vi "_TEST Templates.vi"(4 "error in (no error)":errorcluster) -> (0 "error out":errorcluster)   [LabVIEW 2011]
uses:
  Template Record.ctl
  <vilib>/addons/internet/utils/keyedarr.llb/Keyed Array.ctl
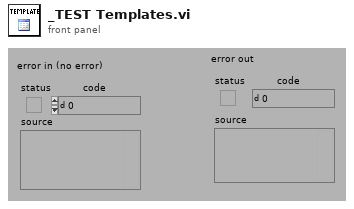
[diagram p1: front panel]
types:
  T1 = typedef "Keyed Array.ctl" = cluster{"keys":string[], "values":string[]}
  T2 = typedef "Template Record.ctl" = cluster{"ixTemplate":i32, "sxTemplateId":string, "sDescription":string, "sCreator":string, "tCreationDate":timestamp, "sModifier":string, "tModifiedDate":timestamp, "sType":string, "sStyle":string, "sFormat":string, "dWidth":dbl, "dHeight":dbl, "sFilename":string, "sScript":string, "sLayout":string, "sEditor":string, "sStyleProcess":string}
  T3 = typedef "Connection Refnum.ctl" = cluster{"Environment Handle":i32, "Connection Handle":i32}
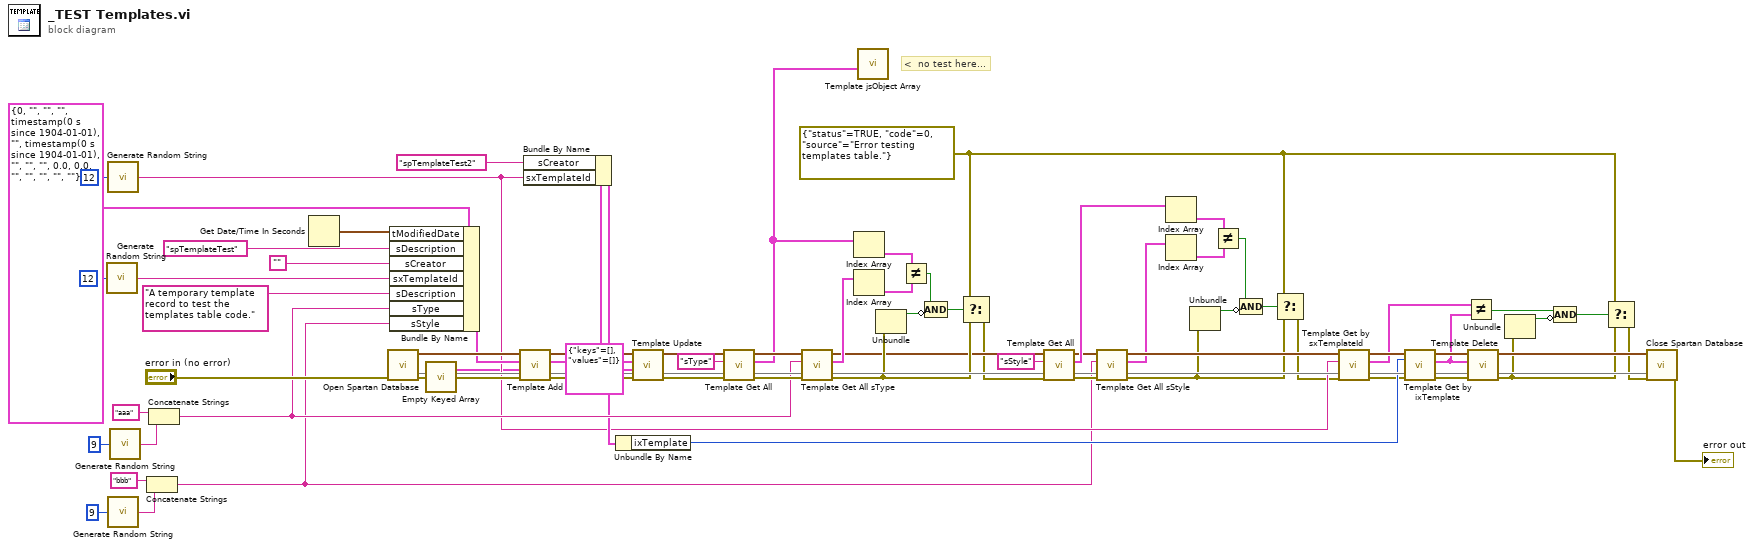
[diagram p0: block diagram]
diagram:
  w19 = errorcluster {"status"=TRUE, "code"=0, "source"="Error testing templates table."} ("t")
  # "<  no test here..."
  n1 = call "Generate Random String.vi"("String Length (5)"=12) -> ("Output String"=w42:string)  [unwired: 4 out]
  n2 = call "Generate Random String.vi"("String Length (5)"=12) -> ("Output String"=w26:string)  [unwired: 4 out]
  n3 = call "Generate Random String.vi"("String Length (5)"=9) -> ("Output String"=w10:string)  [unwired: 4 out]
  n4 = call "Generate Random String.vi"("String Length (5)"=9) -> ("Output String"=w33:string)  [unwired: 4 out]
  n5 = Concatenate Strings("bbb" ("string"), w10) -> (w7:string)
  n6 = Concatenate Strings("aaa" ("string"), w33) -> (w32:string)
  n7 = Get Date/Time In Seconds() -> (seconds since 1Jan1904=w2:timestamp)
  n8 = call "Open Spartan Database.vi"("error in (no error)"="error in (no error)") -> ("error out"=w64:errorcluster, "Connection Refnum"=w66:T3, 4:w71)  [unwired: 1 in, 7 out]
  n9 = Bundle By Name(cluster=T2 {"ixTemplate"=0, "sxTemplateId"="", "sDescription"="", "sCreator"="", "tCreationDate"=timestamp(0 s since 1904-01-01), "sModifier"="", "tModifiedDate"=timestamp(0 s since 1904-01-01), "sType"="", "sStyle"="", "sFormat"="", "dWidth"=0.0, "dHeight"=0.0, "sFilename"="", "sScript"="", "sLayout"="", "sEditor"="", "sStyleProcess"=""} ("Template Record"), "tModifiedDate"=w2, "sDescription"="spTemplateTest", "sCreator"="", "sxTemplateId"=w42, "sDescription"="A temporary template record to test the templates table code.", "sType"=w32, "sStyle"=w7) -> (w39:T2)
  n10 = call "Empty Keyed Array.vi"() -> ("empty keyed array"=w4:T1)  [unwired: 3 out]
  n11 = call "Template Add.vi"("error in (no error)"=w64, "Parameters (empty)"=w4, "Template Record"=w39, "Connection Refnum"=w66) -> ("error out"=w63:errorcluster, "New Template Record"=w62:T2, "Connection Refnum"=w65:T3)  [unwired: 5 out]
  n12 = Bundle By Name(cluster=w62, "sCreator"="spTemplateTest2", "sxTemplateId"=w26) -> (w31:T2)
  n13 = Unbundle By Name(w31) -> ("ixTemplate"=w30:i32)
  n14 = call "Template Update.vi"("error in (no error)"=w63, "Parameters (empty)"=T1 {"keys"=[], "values"=[]}, "Template Record"=w31, "Connection Refnum"=w65) -> ("error out"=w67:errorcluster, "Connection Refnum"=w68:T3)  [unwired: 6 out]
  n15 = call "Template Get All.vi"("error in (no error)"=w67, "Order By (\"sxTemplateId\")"="sType" ("Order By (\"sxTemplateId\")"), "Connection Refnum"=w68) -> ("error out"=w52:errorcluster, "Templates"=w3:T2[], "Connection Refnum"=w53:T3)  [unwired: 6 out]
  n16 = call "Template Get All sType.vi"("error in (no error)"=w52, "sType (\"\")"=w32, "Connection Refnum"=w53) -> ("error out"=w18:errorcluster, "Templates"=w50:T2[], "Connection Refnum"=w17:T3)  [unwired: 6 out]
  n17 = Index Array(array=w3) -> (element=w46:T2)  [unwired: 1 in]
  n18 = Index Array(array=w50) -> (element=w47:T2)  [unwired: 1 in]
  n19 = call "Template jsObject Array.vi"("TEMPLATES (none)"=w3) -> ()  [unwired: 3 in, 8 out]
  n20 = Unbundle(w18) -> ("status"=w48:bool)  [unwired: 2 out]
  n21 = Not Equal?(x=w46, y=w47) -> (x != y?=w45:bool)
  n22 = Compound Arithmetic op=AND(w45, invert w48) -> (w49:bool)
  n23 = Select(t=w19, s=w49, f=w18) -> (s? t:f=w16:errorcluster)
  n24 = call "Template Get All.vi"("error in (no error)"=w16, "Order By (\"sxTemplateId\")"="sStyle" ("Order By (\"sxTemplateId\")"), "Connection Refnum"=w17) -> ("error out"=w14:errorcluster, "Templates"=w15:T2[], "Connection Refnum"=w13:T3)  [unwired: 6 out]
  n25 = call "Template Get All sStyle.vi"("error in (no error)"=w14, "sStyle (\"\")"=w7, "Connection Refnum"=w13) -> ("error out"=w6:errorcluster, "Templates"=w11:T2[], "Connection Refnum"=w12:T3)  [unwired: 6 out]
  n26 = Index Array(array=w15) -> (element=w23:T2)  [unwired: 1 in]
  n27 = Index Array(array=w11) -> (element=w22:T2)  [unwired: 1 in]
  n28 = Unbundle(w6) -> ("status"=w21:bool)  [unwired: 2 out]
  n29 = Not Equal?(x=w23, y=w22) -> (x != y?=w24:bool)
  n30 = Compound Arithmetic op=AND(w24, invert w21) -> (w20:bool)
  n31 = Select(t=w19, s=w20, f=w6) -> (s? t:f=w5:errorcluster)
  n32 = call "Template Get by sxTemplateId.vi"("error in (no error)"=w5, "sxTemplateId (\"\")"=w26, "Connection Refnum"=w12) -> ("error out"=w27:errorcluster, "Template Record"=w28:T2, "Connection Refnum"=w29:T3)  [unwired: 6 out]
  n33 = call "Template Get by ixTemplate.vi"("error in (no error)"=w27, "ixTemplate (0)"=w30, "Connection Refnum"=w29) -> ("error out"=w61:errorcluster, "Template Record"=w59:T2, "Connection Refnum"=w60:T3)  [unwired: 6 out]
  n34 = Not Equal?(x=w28, y=w59) -> (x != y?=w55:bool)
  n35 = call "Template Delete.vi"("error in (no error)"=w61, "Template Record"=w59, "Connection Refnum"=w60) -> ("error out"=w57:errorcluster, "Connection Refnum"=w72:T3)  [unwired: 7 out]
  n36 = Unbundle(w57) -> ("status"=w56:bool)  [unwired: 2 out]
  n37 = Compound Arithmetic op=AND(w55, invert w56) -> (w54:bool)
  n38 = Select(t=w19, s=w54, f=w57) -> (s? t:f=w58:errorcluster)
  n39 = call "Close Spartan Database.vi"("Force Close? (f)"=w71, "error in (no error)"=w58, "Connection Refnum"=w72) -> ("error out"=→"error out":errorcluster)  [unwired: 1 in, 7 out]
